vi "SC TCP Write Data.vi"(6 "timeout ms (25000)":i32, 8 "error in":errorcluster, 10 "Data":string, 11 "TCP Network Connection in":refnum<k5>) -> (0 "error out":errorcluster, 3 "TCP Network Connection out":refnum<k5>)   [LabVIEW 2018]
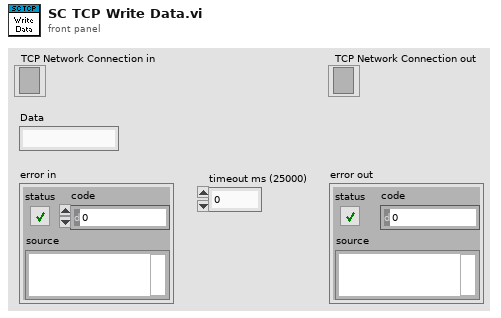
[diagram p1: front panel]
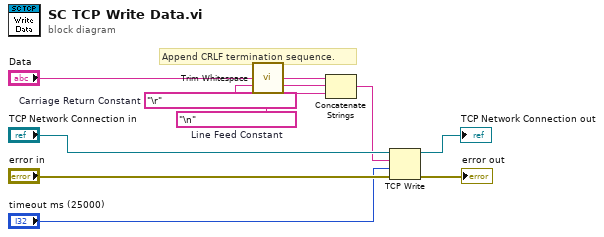
[diagram p0: block diagram]
diagram:
  w1 = "\n"  # Line Feed Constant
  w2 = "\r"  # Carriage Return Constant
  # "Append CRLF termination sequence."
  n1 = call <vilib>:"Trim Whitespace.vi"("string"="Data") -> ("trimmed string"=w3:string)  [unwired: 1 in]
  n2 = Concatenate Strings(w3, w2, w1) -> (w4:string)
  n3 = TCP Write(connection ID="TCP Network Connection in", data in=w4, error in (no error)="error in", 9:"timeout ms (25000)") -> (connection ID out=→"TCP Network Connection out":refnum<k5>, error out=→"error out":errorcluster)  [unwired: 1 out]
